vi "Handle Template.vi"(7 "Processing In":refnum<class "Processing.lvclass">, 8 "error in (no error)":errorcluster, 10 "Path":path, 11 "TemplatedFileServe in":refnum<class "TemplatedFileServe.lvclass">) -> (0 "error out":errorcluster, 2 "Response":refnum<class "Response.lvclass">, 3 "TemplatedFileServe out":refnum<class "TemplatedFileServe.lvclass">, 5 "Processing":refnum<class "Processing.lvclass">)   [LabVIEW 2020, in "HTTP Server.lvlib" / "TemplatedFileServe.lvclass"]
uses:
  TemplatedFileServe.lvclass
  lv-http-util/HTTP Utils/Response/Response.lvclass
  Processing/Processing.lvclass
  TemplateService/TemplateService.lvclass
  C:/dev/lv20CE/relink/lv-http-server/HTTP Server/Service/Service.lvclass
  Processing/Processing.lvclass/Processing.ctl
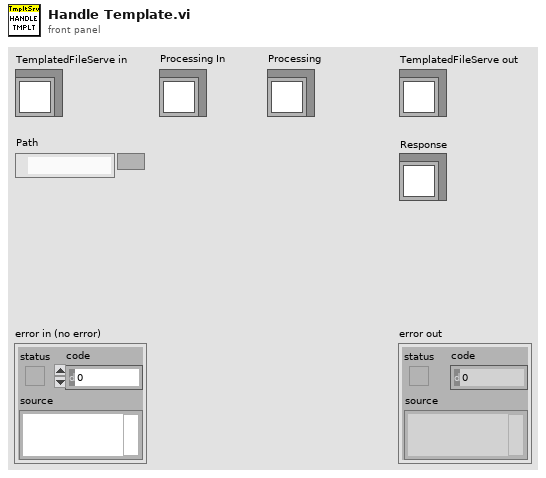
[diagram p1: front panel]
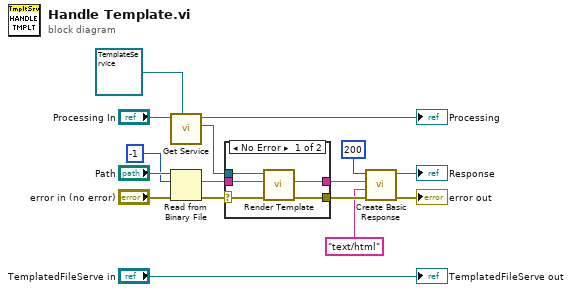
[diagram p0: block diagram]
diagram:
  n1 = call "Get Service.vi"("Service Type"=refnum<class "TemplateService.lvclass"> refnum ("HTTP Server:TemplateService.lvclass"), "Processing in"="Processing In") -> ("Service"=w12:refnum<class "TemplateService.lvclass">, "Processing out"=→"Processing":refnum<class "Processing.lvclass">)  [unwired: 7 in, 1 out]
  n2 = Read from Binary File(8:"error in (no error)", 10:-1 ("count (1)"), 11:"Path") -> (0:w8:errorcluster, 2:w9:string)  [unwired: 3 in, 2 out]
  n3 = case shown="No Error" w8 {
    selector: w8 -> [w19 w22]
    tunnel: w12 -> [w21 _]
    tunnel: w9 -> [w20 _]
    tunnel: [w17 w22] -> w16
    tunnel: [w18 _] -> w6
    frame No Error {
      n4 = call-dynamic "Render Template.vi"("error in (no error)"=w19, "Template"=w20, "TemplateService in"=w21) -> ("error out"=w17:errorcluster, "Output"=w18:string)  [unwired: 6 in, 1 out]
    }
    frame Error {
    }
  }
  n5 = call "Create Basic Response.vi"("error in (no error)"=w16, "Content-Type (text/plain)"="text/html", "Payload"=w6, "Status Code"=u16 200) -> ("error out"=→"error out":errorcluster, "Response out"=→"Response":refnum<class "Response.lvclass">)  [unwired: 6 in]
  "TemplatedFileServe out" <- "TemplatedFileServe in"
